vi "Script Add Custom Error.vi"(4 "Project Reference":refnum<vi>, 5 "Error Code":i32, 6 "Error Description":string, 7 "Error Name":string="TESTING.vi", 8 "error in":errorcluster, 9 "Error Arguments Window Ref":refnum<vi>, 10 "DQMH Lib Ref":refnum<vi>) -> (0 "error out":errorcluster)   [LabVIEW 2020, in "ConstantErrorsMaker.lvlib"]
uses:
  ConstantErrorsMaker.lvlib
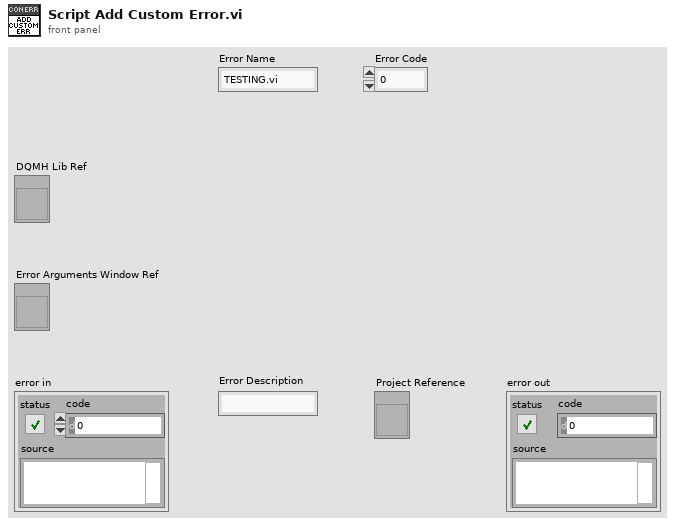
[diagram p1: front panel]
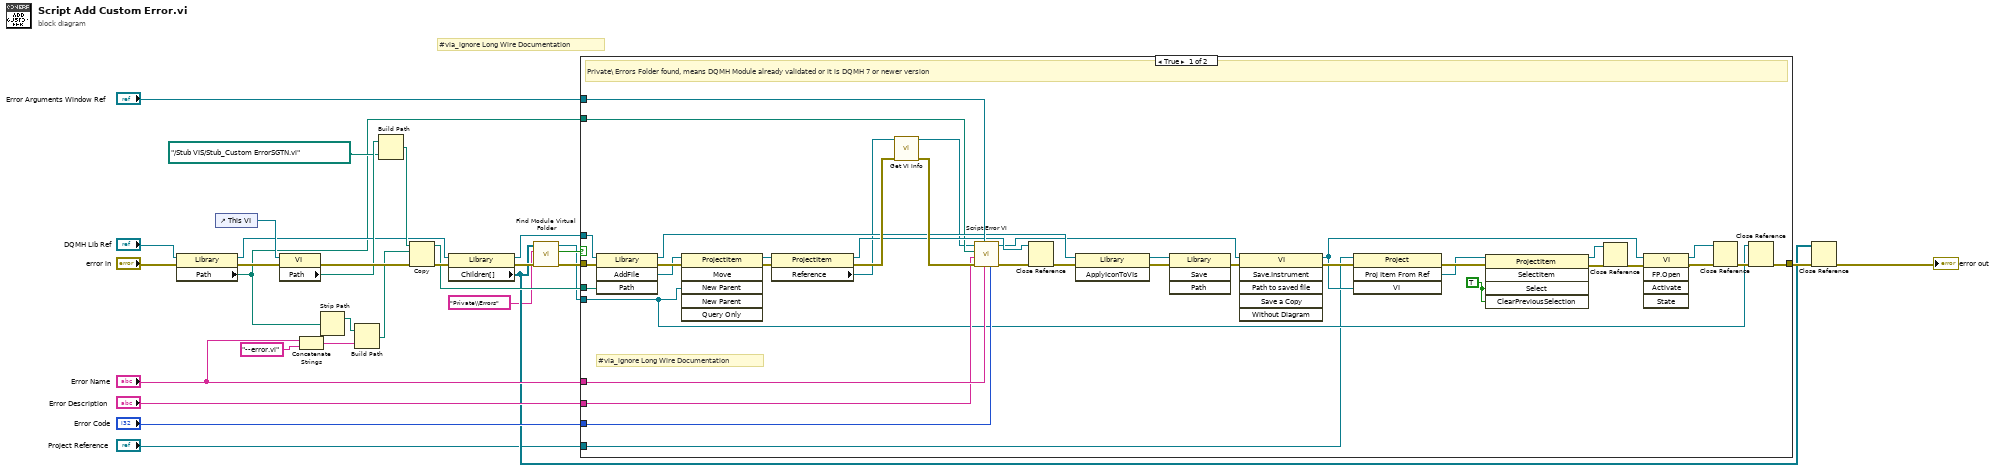
[diagram p0: block diagram]
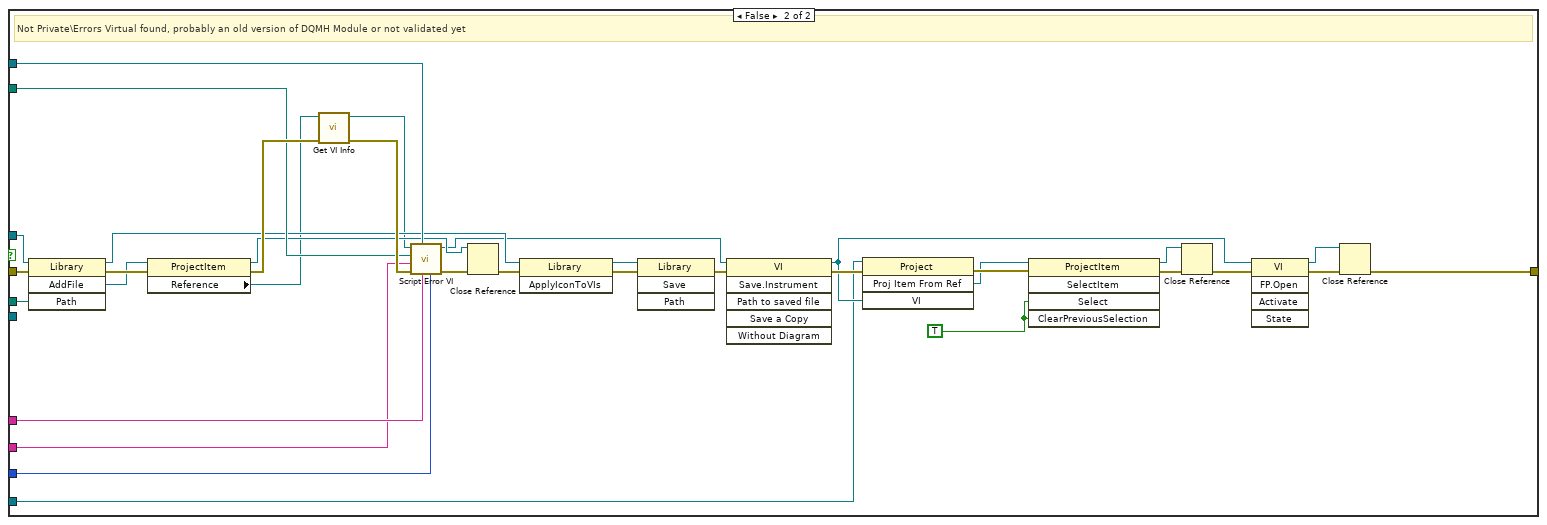
[diagram p2: hidden frame]
diagram:
  # "#via_ignore Long Wire Documentation"
  n1 = property class="Library"(reference="DQMH Lib Ref", error in="error in") -> (reference out=w13:refnum<vi>, error out=w28:errorcluster, "Path"=w11:path)
  n2 = control-ref of="This VI"() -> (w20:refnum<vi>)
  n3 = property class="VI"(reference=w20, error in=w28) -> (error out=w29:errorcluster, "Path"=w19:path)  [unwired: 1 out]
  n4 = Concatenate Strings("Error Name", "--error.vi" ("input 1")) -> (w22:string)
  n5 = Strip Path(path=w11) -> (stripped path=w14:path)  [unwired: 1 out]
  n6 = Build Path(base path=w14, name or relative path=w22) -> (appended path=w21:path)
  n7 = Build Path(base path=w19, name or relative path=path "../Stub VIS/Stub_Custom ErrorSGTN.vi") -> (appended path=w17:path)
  n8 = Copy(8:w29, 10:w21, 11:w17) -> (0:w27:errorcluster, 3:w12:path)  [unwired: 2 in, 1 out]
  n9 = property class="Library"(reference=w13, error in=w27) -> (reference out=w16:refnum<vi>, error out=w24:errorcluster, "Children[]"=w5:refnum<vi>[])
  n10 = call "Find Module Virtual Folder.vi"("error in"=w24, "Virtual Folder"="Private\\Errors", "Children"=w5) -> ("error out"=w23:errorcluster, "Found?"=w4:bool, "ProjectItem out"=w3:refnum<vi>)  [unwired: 6 in]
  n11 = case shown="True" w4 {
    tunnel: [w66 w97] -> w30
    tunnel: w16 -> [w51 w87]
    tunnel: w12 -> [w52 w88]
    tunnel: w11 -> [w33 w85]
    tunnel: "Error Name" -> [w45 w81]
    tunnel: "Error Code" -> [w48 w84]
    tunnel: "Error Arguments Window Ref" -> [w47 w83]
    tunnel: "Error Description" -> [w40 w76]
    tunnel: w3 -> [w39 _]
    tunnel: w23 -> [w60 w91]
    tunnel: "Project Reference" -> [w35 w72]
    frame True {
      w36 = TRUE ("Select")
      # "#via_ignore Long Wire Documentation"
      # "Private\\ Errors Folder found, means DQMH Module already validated or it is DQMH 7 or newer version"
      n12 = invoke class="Library" method="AddFile"(reference=w51, error in=w60, "Path"=w52) -> (reference out=w44:refnum<vi>, error out=w67:errorcluster, "AddFile"=w50:refnum<vi>)  [unwired: 1 in, 1 out]
      n13 = invoke class="ProjectItem" method="Move"(reference=w50, error in=w67, "New Parent"=w39) -> (reference out=w49:refnum<vi>, error out=w68:errorcluster)  [unwired: 3 in, 4 out]
      n14 = property class="ProjectItem"(reference=w49, error in=w68) -> (reference out=w46:refnum<vi>, error out=w54:errorcluster, "Reference"=w32:refnum<vi>)
      n15 = call "Get VI Info.vi"("error in"=w54, "VI in"=w32) -> ("error out"=w53:errorcluster, "VI out"=w31:refnum<vi>)  [unwired: 4 in, 4 out]
      n16 = call "Script Error VI.vi"("Error Code"=w48, "Error Name"=w45, "Error Arguments Window Ref"=w47, "error in"=w53, "Error Description"=w40, "Library Path"=w33, "VI Ref Error in"=w31) -> ("error out"=w56:errorcluster, "Custom Error VI Ref"=w41:refnum<vi>)  [unwired: 3 in]
      n17 = Close Reference(reference=w46, error in (no error)=w56) -> (error out=w65:errorcluster)
      n18 = invoke class="Library" method="ApplyIconToVIs"(reference=w44, error in=w65) -> (reference out=w43:refnum<vi>, error out=w64:errorcluster)  [unwired: 1 in, 1 out]
      n19 = invoke class="Library" method="Save"(reference=w43, error in=w64) -> (error out=w63:errorcluster)  [unwired: 2 in, 3 out]
      n20 = invoke class="VI" method="Save.Instrument"(reference=w41, error in=w63) -> (reference out=w38:refnum<vi>, error out=w59:errorcluster)  [unwired: 4 in, 4 out]
      n21 = invoke class="Project" method="Proj Item From Ref"(reference=w35, error in=w59, "VI"=w38) -> (error out=w58:errorcluster, "ProjItemFromRef"=w37:refnum<vi>)  [unwired: 1 in, 2 out]
      n22 = invoke class="ProjectItem" method="SelectItem"(reference=w37, error in=w58, "Select"=w36, "ClearPreviousSelection"=w36) -> (reference out=w34:refnum<vi>, error out=w57:errorcluster)  [unwired: 1 in, 3 out]
      n23 = Close Reference(reference=w34, error in (no error)=w57) -> (error out=w55:errorcluster)
      n24 = invoke class="VI" method="FP.Open"(reference=w38, error in=w55) -> (reference out=w42:refnum<vi>, error out=w62:errorcluster)  [unwired: 3 in, 3 out]
      n25 = Close Reference(reference=w42, error in (no error)=w62) -> (error out=w61:errorcluster)
      n26 = Close Reference(reference=w39, error in (no error)=w61) -> (error out=w66:errorcluster)
    }
    frame False {
      w74 = TRUE ("Select")
      # "Not Private\\Errors Virtual found, probably an old version of DQMH Module or not validated yet"
      n27 = invoke class="Library" method="AddFile"(reference=w87, error in=w91, "Path"=w88) -> (reference out=w80:refnum<vi>, error out=w102:errorcluster, "AddFile"=w86:refnum<vi>)  [unwired: 1 in, 1 out]
      n28 = property class="ProjectItem"(reference=w86, error in=w102) -> (reference out=w82:refnum<vi>, error out=w90:errorcluster, "Reference"=w69:refnum<vi>)
      n29 = call "Get VI Info.vi"("error in"=w90, "VI in"=w69) -> ("error out"=w89:errorcluster, "VI out"=w70:refnum<vi>)  [unwired: 4 in, 4 out]
      n30 = call "Script Error VI.vi"("Error Code"=w84, "Error Name"=w81, "Error Arguments Window Ref"=w83, "error in"=w89, "Error Description"=w76, "Library Path"=w85, "VI Ref Error in"=w70) -> ("error out"=w93:errorcluster, "Custom Error VI Ref"=w77:refnum<vi>)  [unwired: 3 in]
      n31 = Close Reference(reference=w82, error in (no error)=w93) -> (error out=w101:errorcluster)
      n32 = invoke class="Library" method="ApplyIconToVIs"(reference=w80, error in=w101) -> (reference out=w79:refnum<vi>, error out=w100:errorcluster)  [unwired: 1 in, 1 out]
      n33 = invoke class="Library" method="Save"(reference=w79, error in=w100) -> (error out=w99:errorcluster)  [unwired: 2 in, 3 out]
      n34 = invoke class="VI" method="Save.Instrument"(reference=w77, error in=w99) -> (reference out=w73:refnum<vi>, error out=w95:errorcluster)  [unwired: 4 in, 4 out]
      n35 = invoke class="Project" method="Proj Item From Ref"(reference=w72, error in=w95, "VI"=w73) -> (error out=w96:errorcluster, "ProjItemFromRef"=w75:refnum<vi>)  [unwired: 1 in, 2 out]
      n36 = invoke class="ProjectItem" method="SelectItem"(reference=w75, error in=w96, "Select"=w74, "ClearPreviousSelection"=w74) -> (reference out=w71:refnum<vi>, error out=w94:errorcluster)  [unwired: 1 in, 3 out]
      n37 = Close Reference(reference=w71, error in (no error)=w94) -> (error out=w92:errorcluster)
      n38 = invoke class="VI" method="FP.Open"(reference=w73, error in=w92) -> (reference out=w78:refnum<vi>, error out=w98:errorcluster)  [unwired: 3 in, 3 out]
      n39 = Close Reference(reference=w78, error in (no error)=w98) -> (error out=w97:errorcluster)
    }
  }
  n40 = Close Reference(reference=w5, error in (no error)=w30) -> (error out=→"error out":errorcluster)
